vi "get all subsections.vi"(9 "Item Ref in":T1 format="%.0x", 11 "Child Sections In":T1[](array[typedef]) format="%.0x") -> (1 "Item Ref out":T1 format="%.0x", 3 "Child Sections Out":T1[](array[typedef]) format="%.0x")   [LabVIEW 2018, in "CAN Gateway System Explorer.lvlib"]
uses:
  CAN Gateway System Explorer.lvlib
  <vilib>/NI Veristand/Custom Device API/Custom Device Item Ref.ctl
  <vilib>/NI Veristand/Custom Device API/Custom Device API.lvlib
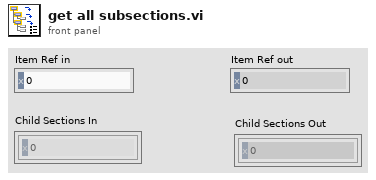
[diagram p1: front panel]
types:
  T1 = typedef "Custom Device API.lvlib/Custom Device Item Ref.ctl" = u64
  T2 = typedef "Custom Device API.lvlib/Custom Device Item Info.ctl" = cluster{"Name":string, "Is Channel":bool, "GUID":string, "Is Waveform":bool}
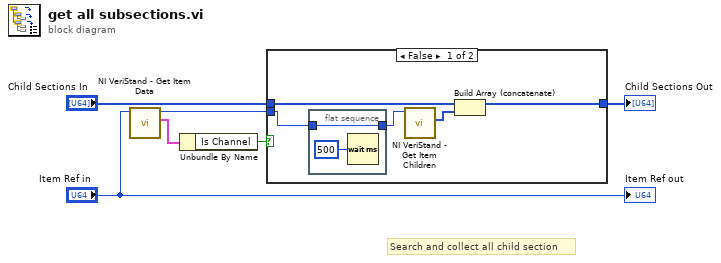
[diagram p0: block diagram]
diagram:
  # "Search and collect all child section"
  n1 = call <vilib>:"NI VeriStand - Get Item Data.vi"("Item Ref in"="Item Ref in") -> ("Item Info"=w4:T2, "Item Ref out"=w6:T1)  [unwired: 7 in, 2 out]
  n2 = Unbundle By Name(w4) -> ("Is Channel"=w5:bool)
  n3 = case shown="False" w5 {
    tunnel: w6 -> [w10 _]
    tunnel: [w8 w14] -> w1
    tunnel: "Child Sections In" -> [w11 w14]
    frame False {
      n4 = flat-sequence {
        tunnel: w10 -> [w12]
        tunnel: [w12] -> w9
        frame #0 {
          n5 = Wait (ms)(milliseconds to wait=u32 500) -> ()  [unwired: 1 out]
        }
      }
      n6 = call <vilib>:"NI VeriStand - Get Item Children.vi"("Item Ref in"=w9) -> ("Child Refs"=w7:T1[])  [unwired: 7 in, 3 out]
      n7 = Build Array (concatenate)(w11, w7) -> (w8:T1[])
    }
    frame True {
    }
  }
  "Child Sections Out" <- w1
  "Item Ref out" <- "Item Ref in"
